vi "StartUp Sequence Open Loop Rev 1.55.vi"() -> ()   [LabVIEW 2017]
panel:
  out "Turbine RPM 2":string
  out "Requested RPM":i32
  out "Waveform Chart":cluster{i32, i32}(graph)
  in  "Set RPM":string
  out "Pump Value 2":string
  in  "Soft Shut Off":bool
  out "Pump Value 1":string
  in  "Send RPM":bool
  in  "Send Command":bool
  in  "Custom Command":string
  out "Startup Success":bool
  in  "Output File":path
  in  "Shut Off":bool
  out "ECU COM Port Out":refnum<visa-resource-name>
  out "Throttle Position":string
  out "Turbine RPM":string
  out "Turbine Temp":string
  out "Error Out":errorcluster
  in  "Error In":errorcluster
  in  "ECU COM Port":refnum<visa-resource-name>
  out "Turbine State":string
  in  "Strt Sqnc":bool
  # "Note: save to a .csv file"
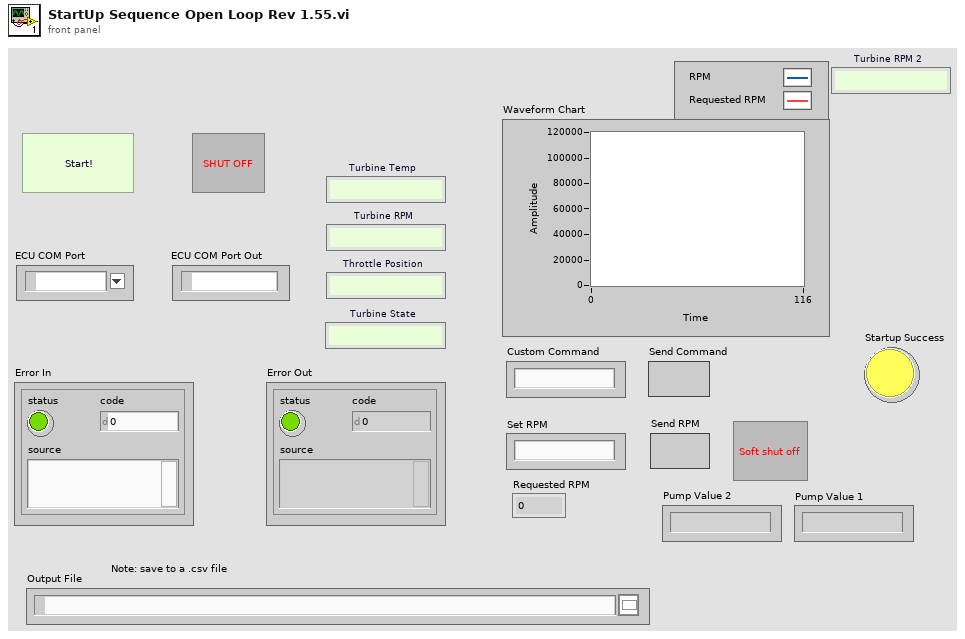
[diagram p1: front panel]
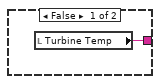
[diagram p4: hidden frame]
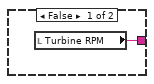
[diagram p5: hidden frame]
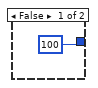
[diagram p7: hidden frame]
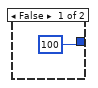
[diagram p8: hidden frame]
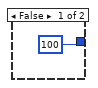
[diagram p9: hidden frame]
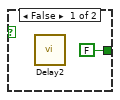
[diagram p11: hidden frame]
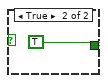
[diagram p12: hidden frame]
diagram:
  w25 = 21 ("Pulse Width")
  w26 = 160 ("Voltage")
  w31 = 16 ("Pulse Width")
  w32 = 160 ("Voltage")
  w22 = 255 ("y")
  w23 = 80 ("y")
  # "Disengage Starter Motor"
  # "Starter Motor 55%"
  # "Start button is inside a while loop that doesn't progess until True"
  # "Fuel Pump Mode 2"
  # "GlowPlugOff"
  # "Start Up\nFuelPumpMode 1"
  # "BurnerValveIgnitionPercent"
  # "If False, each Case structure is set\nto an arbitrary Delay time of 0.2 s"
  # "Each Stage is inside a while loop so that \nthe sequence doesn't progress until True"
  n1 = call "Initialize Com Port.vi"("Error In"="Error In", "ECU COM Port"="ECU COM Port") -> ("Error Out"=w45:errorcluster, "ECU COM Port Out"=w44:refnum<visa-resource-name>)  [unwired: 8 in]
  n2 = while {
    tunnel: w45 -> [w98]
    tunnel: [w98] -> w43
    stop <- "Strt Sqnc" stop-if-true
  }
  n3 = call "Initialize Output File.vi"("error in (no error)"=w43, "File Path Control"="Output File") -> ("error out"=w21:errorcluster)  [unwired: 9 in]
  n4 = flat-sequence {
    tunnel: w21 -> [w100]
    tunnel: [w100] -> w36
    frame #0 {
      n5 = local write "Strt Sqnc"(FALSE ("Strt Sqnc")) -> ()
    }
  }
  n6 = flat-sequence {
    tunnel: [w103] -> w20
    tunnel: w21 -> [w103]
    frame #0 {
      w102 = "0" ("Pump Value 1")
      n7 = local write "Pump Value 2"(w102) -> ()
      n8 = local write "Pump Value 1"(w102) -> ()
    }
  }
  n9 = while {
    tunnel: w20 -> [w124]
    tunnel: w44 -> [w123]
    tunnel: "Output File" -> [w120]
    stop <- w119 continue-if-true
    n10 = call "Get Engine Update.vi"("Error In"=w124, "ECU COM Port"=w123) -> ("Error Out"=w121:errorcluster, "Temperature"=w112:string, "RPMs"=w116:string, "ECU COM Port Out"=w118:refnum<visa-resource-name>)  [unwired: 6 in]
    n11 = call "Time Delay4"() -> ()  [unwired: 11 in, 1 out]
    n12 = call "Safety Check.vi"("Temperature"=w112, "RPMs"=w116) -> ("Safe?"=w119:bool)  [unwired: 9 in]
    n13 = Not Equal?(x=w116, y="") -> (x != y?=w114:bool)
    n14 = Not Equal?(x=w112, y="") -> (x != y?=w111:bool)
    n15 = case shown="False" w119 {
      selector: w119 -> [w129 w131]
      tunnel: w118 -> [w130 _]
      tunnel: [w129 w131] -> w117
      frame False {
        n16 = call "Emergency Shutoff.vi"("ECU COM Port"=w130) -> ()  [unwired: 9 in, 2 out]
      }
      frame True {
      }
    }
    n17 = case shown="True" w114 {
      tunnel: w116 -> [_ w128]
      tunnel: [w127 w128] -> w108
      frame False {
        n18 = local read "Turbine RPM"() -> (w127:string)
      }
      frame True {
        "Turbine RPM" <- w128
      }
    }
    n19 = case shown="True" w111 {
      tunnel: w112 -> [_ w126]
      tunnel: [w125 w126] -> w107
      frame False {
        n20 = local read "Turbine Temp"() -> (w125:string)
      }
      frame True {
        "Turbine Temp" <- w126
      }
    }
    n21 = Not(x=w117) -> (.not. x?=w122:bool)
    n22 = Stop(stop? (T)=w122) -> ()
    n23 = local read "Requested RPM"() -> (w105:i32)
    n24 = local read "Pump Value 2"() -> (w109:string)
    n25 = local read "Pump Value 1"() -> (w110:string)
    n26 = Decimal String To Number(string=w108) -> (number=w106:i32)  [unwired: 2 in, 1 out]
    n27 = Bundle(w106, "Requested RPM"=w105) -> (→"Waveform Chart":cluster{i32, "Requested RPM":i32})  [unwired: 1 in]
    n28 = call "Write Data to Output File.vi"("Pump Value 2"=w109, "Pump Value 1"=w110, "Error In"=w121, "Temperature"=w107, "RPM"=w108, "File Path Control"=w120) -> ()  [unwired: 5 in, 1 out]
  }
  n29 = while {
    tunnel: w44 -> [w133]
    tunnel: w45 -> [_]
    stop <- FALSE stop-if-true
    n30 = case shown="True" "Send Command" {
      tunnel: "Custom Command" -> [_ w137]
      tunnel: w133 -> [_ w136]
      frame False {
      }
      frame True {
        n31 = call "Time Delay3"() -> ()  [unwired: 11 in, 1 out]
        n32 = VISA Write(VISA resource name=w136, write buffer=w137) -> ()  [unwired: 1 in, 3 out]
      }
    }
  }
  n33 = flat-sequence {
    tunnel: w36 -> [_]
    frame #0 {
      n34 = local write "Turbine State"("Initializing Motor") -> ()
    }
  }
  n35 = while {
    tunnel: ["Shut Off"] -> w95
    tunnel: "ECU COM Port" -> [w139]
    stop <- "Shut Off" stop-if-true
    # "Turns off each individual component"
    n36 = case shown="True" "Shut Off" {
      tunnel: w139 -> [_ w143]
      frame False {
      }
      frame True {
        n37 = call "Emergency Shutoff.vi"("ECU COM Port"=w143) -> ("Error Out"=w142:errorcluster)  [unwired: 9 in, 1 out]
        n38 = local write "Output File"(path "" ("Output File")) -> ()
        n39 = flat-sequence {
          tunnel: w142 -> [w144]
          tunnel: [w144] -> _
          frame #0 {
            n40 = local write "Strt Sqnc"(FALSE ("Strt Sqnc")) -> ()
          }
        }
      }
    }
  }
  n41 = call "Set Glow Plug Duty Cycle.vi"("Error In"=w36, "Duty Cycle"=6, "ECU COM Port"=w44) -> ("Error Out"=w88:errorcluster, "ECU COM Port Out"=w85:refnum<visa-resource-name>)  [unwired: 7 in]
  n42 = call "Delay"("error in (no error)"=w88) -> ("error out"=w87:errorcluster)  [unwired: 10 in]
  n43 = call "Set Glow Plug Duty Cycle.vi"("Error In"=w87, "Duty Cycle"=19, "ECU COM Port"=w85) -> ("Error Out"=w86:errorcluster, "ECU COM Port Out"=w81:refnum<visa-resource-name>)  [unwired: 7 in]
  n44 = call "Delay"("error in (no error)"=w86) -> ("error out"=w82:errorcluster)  [unwired: 10 in]
  n45 = call "Set Starter Motor Duty Cycle.vi"("Error In"=w82, "Duty Cycle"=6, "ECU COM Port"=w81) -> ("Error Out"=w80:errorcluster, "ECU COM Port Out"=w78:refnum<visa-resource-name>)  [unwired: 7 in]
  n46 = call "Set Glow Plug Duty Cycle.vi"("Error In"=w80, "Duty Cycle"=15, "ECU COM Port"=w78) -> ("Error Out"=w79:errorcluster, "ECU COM Port Out"=w74:refnum<visa-resource-name>)  [unwired: 7 in]
  n47 = call "Delay"("error in (no error)"=w79) -> ("error out"=w76:errorcluster)  [unwired: 10 in]
  n48 = call "Set Starter Motor Duty Cycle.vi"("Error In"=w76, "Duty Cycle"=4, "ECU COM Port"=w74) -> ("Error Out"=w75:errorcluster, "ECU COM Port Out"=w73:refnum<visa-resource-name>)  [unwired: 7 in]
  n49 = call "Delay"("error in (no error)"=w75) -> ("error out"=w96:errorcluster)  [unwired: 10 in]
  n50 = Stop(stop? (T)=w95) -> ()
  n51 = while {
    tunnel: w96 -> [w148]
    tunnel: w73 -> [w147]
    tunnel: [w147] -> w34
    tunnel: [w148] -> w97
    stop <- w151 stop-if-true
    n52 = local read "Turbine RPM"() -> (w146:string)
    n53 = Decimal String To Number(string=w146) -> (number=w150:i32)  [unwired: 2 in, 1 out]
    n54 = Greater Or Equal?(x=w150, y=3300) -> (x >= y?=w152:bool)
    n55 = case shown="True" w152 {
      tunnel: [FALSE TRUE] -> w151
      frame False {
        n56 = call "Delay2"() -> ()  [unwired: 11 in, 1 out]
      }
      frame True {
      }
    }
  }
  n57 = flat-sequence {
    tunnel: w96 -> [_]
    frame #0 {
      n58 = local write "Turbine State"("Stage1 Check RPM") -> ()
    }
  }
  n59 = call "CmdSeparator7"("error in (no error)"=w97) -> ("error out"=w30:errorcluster)  [unwired: 10 in]
  n60 = call "Set Pump Fow Rate.vi"("Error In"=w30, "Pulse Width"=w31, "Voltage"=w32, "ECU COM Port"=w34) -> ("Error Out"=w35:errorcluster, "ECU COM Port Out"=w33:refnum<visa-resource-name>)  [unwired: 6 in]
  n61 = flat-sequence {
    tunnel: w32 -> [w157]
    tunnel: w31 -> [w156]
    tunnel: w30 -> [_]
    frame #0 {
      n62 = Number To Decimal String(number=w156) -> (decimal integer string=w158:string)  [unwired: 1 in]
      n63 = Number To Decimal String(number=w157) -> (decimal integer string=w159:string)  [unwired: 1 in]
      n64 = local write "Pump Value 2"(w158) -> ()
      n65 = local write "Pump Value 1"(w159) -> ()
    }
  }
  n66 = call "CmdSeparator2"("error in (no error)"=w35) -> ("error out"=w72:errorcluster)  [unwired: 10 in]
  n67 = call "Set Burner Valve Percent.vi"("Error In"=w72, "Percent"=10, "ECU COM Port"=w33) -> ("Error Out"=w71:errorcluster, "ECU COM Port Out"=w18:refnum<visa-resource-name>)  [unwired: 7 in]
  n68 = call "CmdSeparator"("error in (no error)"=w71) -> ("error out"=w17:errorcluster)  [unwired: 10 in]
  n69 = for {
    N: 8 -> [_]
    shift-right: [w165] -> _
    shift-left: 27 ("Percent") -> [w167]
    tunnel: w18 -> [w164]
    tunnel: w17 -> [w163]
    tunnel: [w161] -> w15
    tunnel: [w160] -> w14
    n70 = Add(x=w167, y=4 ("Percent")) -> (x+y=w165:i32)
    n71 = call "Set Burner Valve Percent.vi"("Error In"=w163, "Percent"=w165, "ECU COM Port"=w164) -> ("Error Out"=w162:errorcluster, "ECU COM Port Out"=w160:refnum<visa-resource-name>)  [unwired: 7 in]
    n72 = call "CmdSeparator4"("error in (no error)"=w162) -> ("error out"=w161:errorcluster)  [unwired: 10 in]
  }
  n73 = flat-sequence {
    tunnel: w15 -> [_]
    frame #0 {
      n74 = local write "Turbine State"("Stage2 Check Temp.") -> ()
    }
  }
  n75 = while {
    tunnel: [w169] -> _
    tunnel: w15 -> [w171]
    tunnel: [w169] -> w12
    tunnel: [w171] -> w13
    tunnel: w14 -> [w169]
    stop <- w174 stop-if-true
    # "Stage2Temp(C)"
    n76 = local read "Turbine Temp"() -> (w170:string)
    n77 = Decimal String To Number(string=w170) -> (number=w172:i32)  [unwired: 2 in, 1 out]
    n78 = Greater Or Equal?(x=w172, y=90) -> (x >= y?=w175:bool)
    n79 = case shown="False" w175 {
      tunnel: [FALSE TRUE] -> w174
      frame False {
        n80 = call "Delay3"() -> ()  [unwired: 11 in, 1 out]
      }
      frame True {
      }
    }
  }
  n81 = call "Set Glow Plug Duty Cycle.vi"("Error In"=w13, "Duty Cycle"=0, "ECU COM Port"=w12) -> ("Error Out"=w66:errorcluster, "ECU COM Port Out"=w27:refnum<visa-resource-name>)  [unwired: 7 in]
  n82 = call "CmdSeparator3"("error in (no error)"=w66) -> ("error out"=w24:errorcluster)  [unwired: 10 in]
  n83 = call "Set Pump Fow Rate.vi"("Error In"=w24, "Pulse Width"=w25, "Voltage"=w26, "ECU COM Port"=w27) -> ("Error Out"=w29:errorcluster, "ECU COM Port Out"=w28:refnum<visa-resource-name>)  [unwired: 6 in]
  n84 = call "Set Burner Valve Percent.vi"("Error In"=w29, "Percent"=80, "ECU COM Port"=w28) -> ("Error Out"=w63:errorcluster, "ECU COM Port Out"=w64:refnum<visa-resource-name>)  [unwired: 7 in]
  n85 = flat-sequence {
    tunnel: w26 -> [w179]
    tunnel: w25 -> [w178]
    tunnel: w24 -> [_]
    frame #0 {
      n86 = Number To Decimal String(number=w178) -> (decimal integer string=w180:string)  [unwired: 1 in]
      n87 = Number To Decimal String(number=w179) -> (decimal integer string=w181:string)  [unwired: 1 in]
      n88 = local write "Pump Value 2"(w180) -> ()
      n89 = local write "Pump Value 1"(w181) -> ()
    }
  }
  n90 = call "CmdSeparator18"("error in (no error)"=w63) -> ("error out"=w62:errorcluster)  [unwired: 10 in]
  n91 = call "Set Fuel Valve Percent.vi"("Error In"=w62, "Percent"=12, "ECU COM Port"=w64) -> ("Error Out"=w61:errorcluster, "ECU COM Port Out"=w65:refnum<visa-resource-name>)  [unwired: 7 in]
  n92 = call "CmdSeparator16"("error in (no error)"=w61) -> ("error out"=w94:errorcluster)  [unwired: 10 in]
  n93 = for {
    N: 4 -> [_]
    tunnel: [w182] -> _
    tunnel: [w196] -> _
    tunnel: w65 -> [w188]
    tunnel: w94 -> [w189]
    shift-right: [w187] -> w57
    shift-left: 12 -> [w193]
    shift-right: [w184] -> _
    shift-left: 80 -> [w190]
    tunnel: [w196] -> w55 mode=indexing
    tunnel: [w182] -> w58 mode=indexing
    n94 = Less?(x=w193, y=100) -> (x < y?=w194:bool)
    n95 = Less?(x=w190, y=100) -> (x < y?=w191:bool)
    n96 = case shown="True" w191 {
      tunnel: w190 -> [_ w200]
      tunnel: [100 w198] -> w184
      frame False {
      }
      frame True {
        n97 = Add(x=w200, y=5) -> (x+y=w198:i32)
      }
    }
    n98 = case shown="True" w194 {
      tunnel: w193 -> [_ w204]
      tunnel: [100 w202] -> w187
      frame False {
      }
      frame True {
        n99 = Add(x=w204, y=6) -> (x+y=w202:i32)
      }
    }
    n100 = call "Set Fuel Valve Percent.vi"("Error In"=w189, "Percent"=w187, "ECU COM Port"=w188) -> ("Error Out"=w186:errorcluster, "ECU COM Port Out"=w183:refnum<visa-resource-name>)  [unwired: 7 in]
    n101 = call "Set Burner Valve Percent.vi"("Error In"=w186, "Percent"=w184, "ECU COM Port"=w183) -> ("Error Out"=w185:errorcluster, "ECU COM Port Out"=w182:refnum<visa-resource-name>)  [unwired: 7 in]
    n102 = call "CmdSeparator17"("error in (no error)"=w185) -> ("error out"=w196:errorcluster)  [unwired: 10 in]
  }
  n103 = flat-sequence {
    tunnel: w55 -> [_]
    frame #0 {
      n104 = local write "Turbine State"("Pump Ramp Up") -> ()
    }
  }
  n105 = for {
    N: 10 -> [_]
    tunnel: [w212] -> w47
    tunnel: [w223] -> w48
    shift-right: [w219] -> _
    shift-left: w57 -> [w220]
    tunnel: w55 -> [w216] mode=indexing
    tunnel: w58 -> [w215] mode=indexing
    shift-right: [w208] -> _
    shift-left: 21 -> [w209]
    w207 = 160 ("y")
    n106 = Less?(x=w220, y=100) -> (x < y?=w221:bool)
    n107 = Add(x=w209, y=1) -> (x+y=w208:i32)
    n108 = case shown="True" w221 {
      tunnel: w220 -> [_ w231]
      tunnel: [100 w229] -> w219
      frame False {
      }
      frame True {
        n109 = Add(x=w231, y=5) -> (x+y=w229:i32)
      }
    }
    n110 = call "Set Fuel Valve Percent.vi"("Error In"=w216, "Percent"=w219, "ECU COM Port"=w215) -> ("Error Out"=w218:errorcluster, "ECU COM Port Out"=w217:refnum<visa-resource-name>)  [unwired: 7 in]
    n111 = call "Set Burner Valve Percent.vi"("Error In"=w218, "Percent"=100 ("y"), "ECU COM Port"=w217) -> ("Error Out"=w206:errorcluster, "ECU COM Port Out"=w213:refnum<visa-resource-name>)  [unwired: 7 in]
    n112 = call "Set Pump Fow Rate.vi"("Error In"=w206, "Pulse Width"=w208, "Voltage"=w207, "ECU COM Port"=w213) -> ("Error Out"=w211:errorcluster, "ECU COM Port Out"=w212:refnum<visa-resource-name>)  [unwired: 6 in]
    n113 = flat-sequence {
      tunnel: w207 -> [w225]
      tunnel: w208 -> [w224]
      tunnel: w206 -> [_]
      frame #0 {
        n114 = Number To Decimal String(number=w224) -> (decimal integer string=w226:string)  [unwired: 1 in]
        n115 = Number To Decimal String(number=w225) -> (decimal integer string=w227:string)  [unwired: 1 in]
        n116 = local write "Pump Value 2"(w226) -> ()
        n117 = local write "Pump Value 1"(w227) -> ()
      }
    }
    n118 = call "CmdSeparator20"("error in (no error)"=w211) -> ("error out"=w223:errorcluster)  [unwired: 10 in]
  }
  n119 = call "Set Starter Motor Duty Cycle.vi"("Error In"=w48, "Duty Cycle"=11, "ECU COM Port"=w47) -> ("Error Out"=w10:errorcluster, "ECU COM Port Out"=w11:refnum<visa-resource-name>)  [unwired: 7 in]
  n120 = flat-sequence {
    tunnel: w10 -> [_]
    frame #0 {
      n121 = local write "Turbine State"("Secondary Pump Ramp Up") -> ()
    }
  }
  n122 = while {
    tunnel: w11 -> [w237]
    tunnel: w10 -> [w236]
    tunnel: [w235] -> w9
    tunnel: [w234] -> w8
    stop <- w240 stop-if-true
    w239 = 160 ("y")
    n123 = local read "Turbine RPM"() -> (w246:string)
    n124 = Decimal String To Number(string=w246) -> (number=w242:i32)  [unwired: 2 in, 1 out]
    n125 = Multiply(x=w242, y=0.0008) -> (x*y=w244:dbl)
    n126 = call "Set Fuel Valve Percent.vi"("Error In"=w236, "Percent"=100 ("y"), "ECU COM Port"=w237) -> ("Error Out"=w251:errorcluster, "ECU COM Port Out"=w250:refnum<visa-resource-name>)  [unwired: 7 in]
    n127 = Add(x=w244, y=14.537) -> (x+y=w238:dbl)
    n128 = call "Set Burner Valve Percent.vi"("Error In"=w251, "Percent"=0 ("y"), "ECU COM Port"=w250) -> ("Error Out"=w247:errorcluster, "ECU COM Port Out"=w248:refnum<visa-resource-name>)  [unwired: 7 in]
    n129 = call "Set Pump Fow Rate.vi"("Error In"=w247, "Pulse Width"=w238, "Voltage"=w239, "ECU COM Port"=w248) -> ("Error Out"=w233:errorcluster, "ECU COM Port Out"=w235:refnum<visa-resource-name>)  [unwired: 6 in]
    n130 = call "CmdSeparator5"("error in (no error)"=w233) -> ("error out"=w234:errorcluster)  [unwired: 10 in]
    n131 = flat-sequence {
      tunnel: w239 -> [w255]
      tunnel: w238 -> [w254]
      tunnel: [w253] -> _
      tunnel: w233 -> [w253]
      frame #0 {
        n132 = Number To Decimal String(number=w254) -> (decimal integer string=w256:string)  [unwired: 1 in]
        n133 = Number To Decimal String(number=w255) -> (decimal integer string=w257:string)  [unwired: 1 in]
        n134 = local write "Pump Value 2"(w256) -> ()
        n135 = local write "Pump Value 1"(w257) -> ()
      }
    }
    n136 = Greater Or Equal?(x=w242, y=30000) -> (x >= y?=w240:bool)
  }
  n137 = call "Set Pump Fow Rate.vi"("Error In"=w8, "Pulse Width"=w22, "Voltage"=w23, "ECU COM Port"=w9) -> ("Error Out"=w54:errorcluster, "ECU COM Port Out"=w53:refnum<visa-resource-name>)  [unwired: 6 in]
  n138 = flat-sequence {
    tunnel: w23 -> [w260]
    tunnel: w22 -> [w259]
    tunnel: [w258] -> _
    tunnel: w8 -> [w258]
    frame #0 {
      n139 = Number To Decimal String(number=w259) -> (decimal integer string=w261:string)  [unwired: 1 in]
      n140 = Number To Decimal String(number=w260) -> (decimal integer string=w262:string)  [unwired: 1 in]
      n141 = local write "Pump Value 2"(w261) -> ()
      n142 = local write "Pump Value 1"(w262) -> ()
    }
  }
  n143 = while {
    tunnel: w54 -> [w264]
    tunnel: w53 -> [w263]
    tunnel: [w264] -> w50
    tunnel: [w263] -> w52
    stop <- w265 stop-if-true
    n144 = local read "Turbine RPM"() -> (w268:string)
    n145 = Decimal String To Number(string=w268) -> (number=w267:i32)  [unwired: 2 in, 1 out]
    n146 = Greater?(x=w267, y=44000) -> (0:w265:bool)
  }
  n147 = flat-sequence {
    tunnel: w50 -> [_]
    frame #0 {
      n148 = local write "Turbine State"("Acheived Idle RPM!") -> ()
    }
  }
  n149 = call "Set Starter Motor Duty Cycle.vi"("Error In"=w50, "Duty Cycle"=0, "ECU COM Port"=w52) -> ("Error Out"=w41:errorcluster, "ECU COM Port Out"=w40:refnum<visa-resource-name>)  [unwired: 7 in]
  n150 = flat-sequence {
    tunnel: w41 -> [_]
    frame #0 {
      "Startup Success" <- TRUE
    }
  }
  n151 = while {
    tunnel: w40 -> [w284]
    tunnel: [w283] -> w38
    tunnel: [w282] -> w39
    tunnel: w41 -> [w281]
    stop <- "Soft Shut Off" stop-if-true
    # "NOTE:\nThere are data entry limits\non this input. These may need\nto be deleted in the future"
    n152 = Decimal String To Number(string="Set RPM") -> (number=w272:i32)  [unwired: 2 in, 1 out]
    n153 = Less?(x=w272, y=135000) -> (x < y?=w278:bool)
    n154 = Greater?(x=w272, y=44000) -> (0:w273:bool)
    n155 = And(x=w273, y=w278) -> (x .and. y?=w276:bool)
    n156 = call "Time Delay"() -> ()  [unwired: 11 in, 1 out]
    n157 = And(x=w276, y="Send RPM") -> (x .and. y?=w274:bool)
    n158 = case shown="True" w274 {
      tunnel: w284 -> [w285 w295]
      tunnel: w281 -> [w286 w294]
      tunnel: [w285 w293] -> w283
      tunnel: [w286 w292] -> w282
      tunnel: w272 -> [_ w287]
      frame False {
      }
      frame True {
        n159 = call "RPM to Fuel Flow.vi"("Requested RPM"=w287) -> ("Fuel Pump Value 1"=w288:i32)  [unwired: 10 in]
        n160 = call "Set Pump Fow Rate.vi"("Error In"=w294, "Pulse Width"=255, "Voltage"=w288, "ECU COM Port"=w295) -> ("Error Out"=w292:errorcluster, "ECU COM Port Out"=w293:refnum<visa-resource-name>)  [unwired: 6 in]
        n161 = Number To Decimal String(number=w288) -> (decimal integer string=→"Pump Value 1":string)  [unwired: 1 in]
        n162 = local write "Pump Value 2"("255" ("Pump Value 2")) -> ()
        "Requested RPM" <- w287
      }
    }
  }
  n163 = call "Emergency Shutoff.vi"("Error In"=w39, "ECU COM Port"=w38) -> ("Error Out"=w37:errorcluster, "ECU COM Port Out"=w6:refnum<visa-resource-name>)  [unwired: 8 in]
  n164 = flat-sequence {
    tunnel: w37 -> [w297]
    tunnel: [w297] -> w7
    frame #0 {
      w296 = "0"
      n165 = local write "Pump Value 1"(w296) -> ()
      n166 = local write "Pump Value 2"(w296) -> ()
    }
  }
  n167 = while {
    tunnel: w7 -> [w303]
    tunnel: w6 -> [w300]
    tunnel: [w298] -> w5
    tunnel: [w299] -> w4
    stop <- w304 stop-if-true
    n168 = while {
      tunnel: [w309] -> w302
      tunnel: w303 -> [w309]
      stop <- w312 stop-if-true
      n169 = local read "Turbine RPM"() -> (w313:string)
      n170 = Decimal String To Number(string=w313) -> (number=w310:i32)  [unwired: 2 in, 1 out]
      n171 = Less?(x=30000, y=w310) -> (x < y?=w312:bool)
    }
    n172 = local read "Turbine Temp"() -> (w307:string)
    n173 = Decimal String To Number(string=w307) -> (number=w306:i32)  [unwired: 2 in, 1 out]
    n174 = flat-sequence {
      tunnel: w298 -> [_]
      frame #0 {
        n175 = local write "Turbine State"("Cooling Down") -> ()
      }
    }
    n176 = call "Set Starter Motor Duty Cycle.vi"("Error In"=w302, "Duty Cycle"=4, "ECU COM Port"=w300) -> ("Error Out"=w298:errorcluster, "ECU COM Port Out"=w299:refnum<visa-resource-name>)  [unwired: 7 in]
    n177 = Greater?(x=w306, y=100) -> (0:w304:bool)
  }
  n178 = flat-sequence {
    tunnel: w1 -> [_]
    frame #0 {
      n179 = local write "Turbine State"("Off") -> ()
    }
  }
  n180 = call "Set Starter Motor Duty Cycle.vi"("Error In"=w5, "Duty Cycle"=0, "ECU COM Port"=w4) -> ("Error Out"=w1:errorcluster, "ECU COM Port Out"=→"ECU COM Port Out":refnum<visa-resource-name>)  [unwired: 7 in]
  "Error Out" <- w1
